vi "Win Host - Run List Manager.vi"(5 "Coords":T1, 6 "Reporting?":bool, 7 "Command":T2, 8 "error in (no error)":errorcluster, 9 "All? IN":bool, 10 "Item Names":string[](array[string]), 11 "ListBox in":refnum<vi>) -> (0 "error out":errorcluster, 1 "All? OUT":bool, 2 "Selected Runs?":bool[](array[boolean]), 4 "Item Names Out":string[](array[string]))   [LabVIEW 2024]
uses:
  Controls/Run Listbox Command.ctl
  <vilib>/Utility/miscctls.llb/LVPoint32TypeDef.ctl
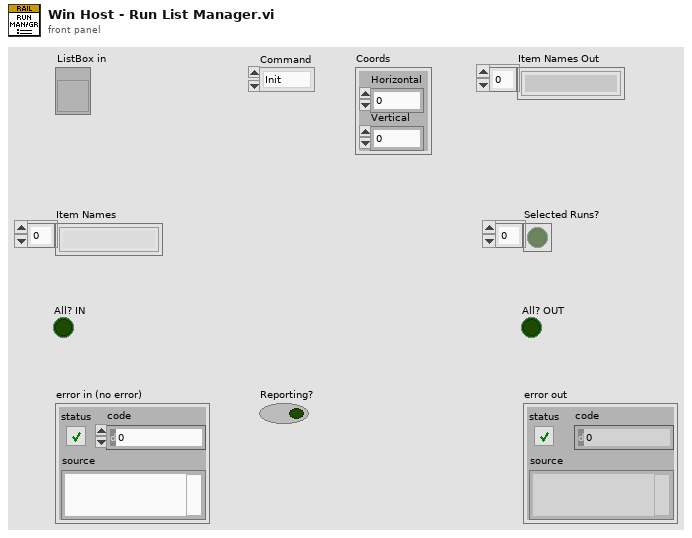
[diagram p1: front panel]
types:
  T1 = typedef "LVPoint32TypeDef.ctl" = cluster{"Horizontal":i32, "Vertical":i32}
  T2 = typedef "Run Listbox Command.ctl" = enum16{"Init", "Item Names", "Update", "Update All", "Get Selections", "Clear"}
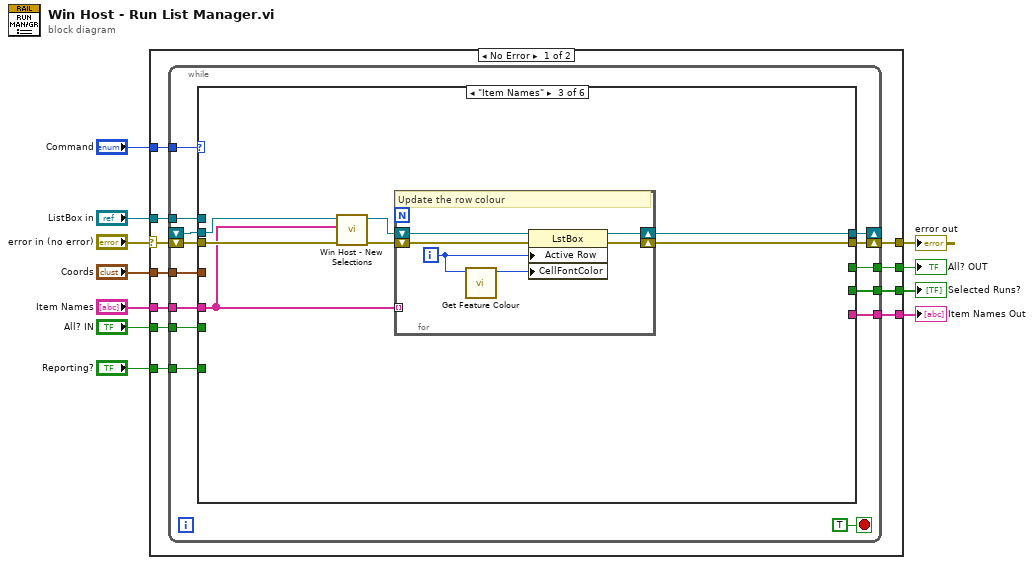
[diagram p0: block diagram]
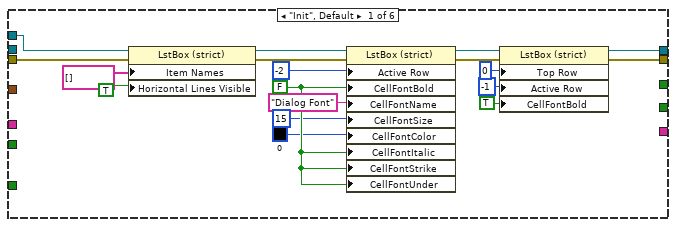
[diagram p2: hidden frame]
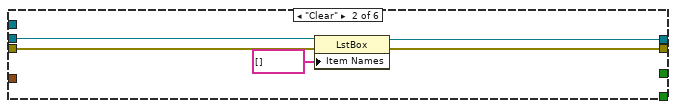
[diagram p3: hidden frame]
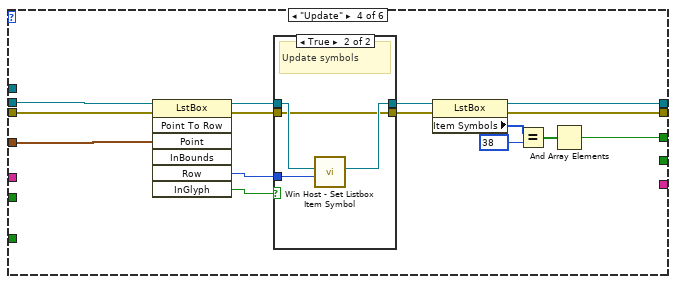
[diagram p4: hidden frame]
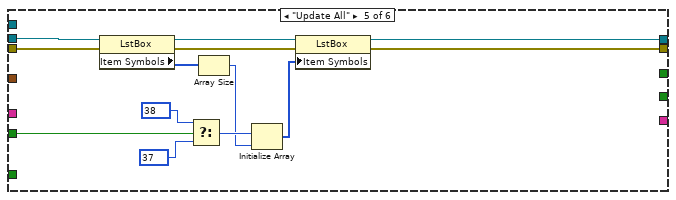
[diagram p6: hidden frame]
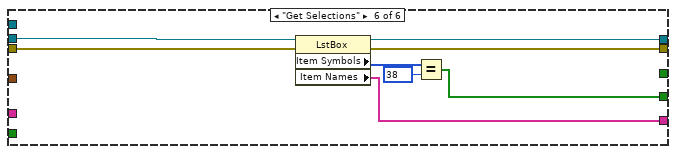
[diagram p7: hidden frame]
diagram:
  n1 = case shown="No Error" "error in (no error)" {
    selector: "error in (no error)" -> [w21 w115]
    tunnel: [w22 w115] -> w11
    tunnel: "Command" -> [w20 _]
    tunnel: "Coords" -> [w19 _]
    tunnel: "Item Names" -> [w18 _]
    tunnel: "ListBox in" -> [w17 _]
    tunnel: [w16 _] -> w5
    tunnel: "All? IN" -> [w15 _]
    tunnel: [w14 _] -> w3
    tunnel: "Reporting?" -> [w13 _]
    tunnel: [w12 _] -> w1
    frame No Error {
      n2 = while {
        shift-right: [w36] -> w22
        shift-left: w21 -> [w34]
        tunnel: w20 -> [w32]
        tunnel: w19 -> [w26]
        tunnel: w18 -> [w29]
        shift-right: [w30] -> _
        shift-left: _ -> [w35]
        tunnel: w17 -> [w31]
        tunnel: [w28] -> w16
        tunnel: w15 -> [w27]
        tunnel: [w25] -> w14
        tunnel: w13 -> [w24]
        tunnel: [w23] -> w12
        stop <- TRUE stop-if-true
        n3 = case shown="\"Item Names\"" w32 {
          tunnel: [w54 w59 w61 w74 w106 w114] -> w36
          tunnel: w35 -> [_ w56 w65 w87 w103 w111]
          tunnel: w34 -> [w39 w57 w66 w86 w104 w112]
          tunnel: w31 -> [w38 _ _ _ _ _]
          tunnel: [w37 w58 w62 w73 w105 w113] -> w30
          tunnel: w29 -> [_ _ w60 _ _ _]
          tunnel: [_ _ _ w77 _ _] -> w28
          tunnel: w27 -> [_ _ _ _ w94 _]
          tunnel: w26 -> [_ _ _ w81 _ _]
          tunnel: [_ _ _ _ _ w108] -> w25
          tunnel: w24 -> [_ _ _ _ _ _]
          tunnel: [_ _ _ _ _ w107] -> w23
          frame "Init", Default {
            w49 = FALSE ("Active Row:Cell Font:Bold")
            n4 = property class="LstBox (strict)"(reference=w38, error in=w39, "Item Names"=string[] [], "Horizontal Lines Visible"=TRUE ("Visible Items:Horizontal Lines Visible")) -> (reference out=w43:refnum<vi>, error out=w45:errorcluster)
            n5 = property on="Property Node" class="LstBox (strict)"(reference=w43, error in=w45, "Active Row"=-2 ("Active Row:Active Row Number"), "CellFontBold"=w49, "CellFontName"="Dialog Font" ("Active Row:Cell Font:Name"), "CellFontSize"=u32 15 ("Active Row:Cell Font:Size"), "CellFontColor"=u32 0, "CellFontItalic"=w49, "CellFontStrike"=w49, "CellFontUnder"=w49) -> (reference out=w53:refnum<vi>, error out=w52:errorcluster)
            n6 = property class="LstBox (strict)"(reference=w53, error in=w52, "Top Row"=0, "Active Row"=-1 ("Active Row:Active Row Number"), "CellFontBold"=TRUE ("Active Row:Cell Font:Bold")) -> (reference out=w37:refnum<vi>, error out=w54:errorcluster)
          }
          frame "Clear" {
            n7 = property class="LstBox"(reference=w56, error in=w57, "Item Names"=string[] []) -> (reference out=w58:refnum<vi>, error out=w59:errorcluster)
          }
          frame "Item Names" {
            n8 = call "Win Host - New Selections.vi"("error in (no error)"=w66, "New Item Names"=w60, "ListBox in"=w65) -> ("error out"=w64:errorcluster, "ListBox out"=w63:refnum<vi>)  [unwired: 7 in]
            n9 = for {
              shift-right: [w69] -> w61
              shift-left: w64 -> [w72]
              shift-right: [w70] -> w62
              shift-left: w63 -> [w71]
              tunnel: w60 -> [_] mode=indexing
              i -> [w67]
              # "Update the row colour"
              n10 = call "Get Feature Colour.vi"("Feature Type"=w67) -> ("color"=w68:u32)  [unwired: 10 in]
              n11 = property class="LstBox"(reference=w71, error in=w72, "Active Row"=w67, "CellFontColor"=w68) -> (reference out=w70:refnum<vi>, error out=w69:errorcluster)
            }
          }
          frame "Update" {
            n12 = invoke class="LstBox" method="Point To Row"(reference=w87, error in=w86, "Point"=w81) -> (reference out=w83:refnum<vi>, error out=w85:errorcluster, "Row"=w84:i32, "InGlyph"=w82:bool)  [unwired: 4 in, 3 out]
            n13 = case shown="True" w82 {
              tunnel: w85 -> [w88 w90]
              tunnel: w84 -> [_ w93]
              tunnel: w83 -> [w89 w92]
              tunnel: [w89 w91] -> w76
              tunnel: [w88 w90] -> w75
              frame False {
                # "Do nothing..."
              }
              frame True {
                # "Update symbols"
                n14 = call "Win Host - Set Listbox Item Symbol.vi"("Row"=w93, "Listbox"=w92) -> ("dup Listboc"=w91:refnum<vi>)  [unwired: 6 in]
              }
            }
            n15 = property class="LstBox"(reference=w76, error in=w75) -> (reference out=w73:refnum<vi>, error out=w74:errorcluster, "Item Symbols"=w79:i32[])
            n16 = Equal?(x=w79, y=38) -> (x = y?=w80:bool[])
            n17 = And Array Elements(Boolean array=w80) -> (logical AND=w77:bool)
          }
          frame "Update All" {
            n18 = property class="LstBox"(reference=w103, error in=w104) -> (reference out=w101:refnum<vi>, error out=w102:errorcluster, "Item Symbols"=w100:i32[])
            n19 = Select(t=38, s=w94, f=37) -> (s? t:f=w99:i32)
            n20 = Array Size(array=w100) -> (size(s)=w96:i32)
            n21 = Initialize Array(w99, w96) -> (w95:i32[])
            n22 = property class="LstBox"(reference=w101, error in=w102, "Item Symbols"=w95) -> (reference out=w105:refnum<vi>, error out=w106:errorcluster)
          }
          frame "Get Selections" {
            n23 = property class="LstBox"(reference=w111, error in=w112) -> (reference out=w113:refnum<vi>, error out=w114:errorcluster, "Item Symbols"=w110:i32[], "Item Names"=w107:string[])
            n24 = Equal?(x=w110, y=38) -> (x = y?=w108:bool[])
          }
        }
      }
    }
    frame Error {
    }
  }
  "error out" <- w11
  "All? OUT" <- w5
  "Selected Runs?" <- w3
  "Item Names Out" <- w1
